vi "Tag Metadata Remove Group 01.vi"(0 "Tags Array":string[][](array[string]), 7 "Boolean Refs Array":refnum<vi>[](array[refnum]), 11 "Group Index":i32) -> (4 "Updated Tag Array":string[][](array[string]), 8 "Update Index":i32, 15 "Current Tags":string[][](array[string]))   [LabVIEW 2020]
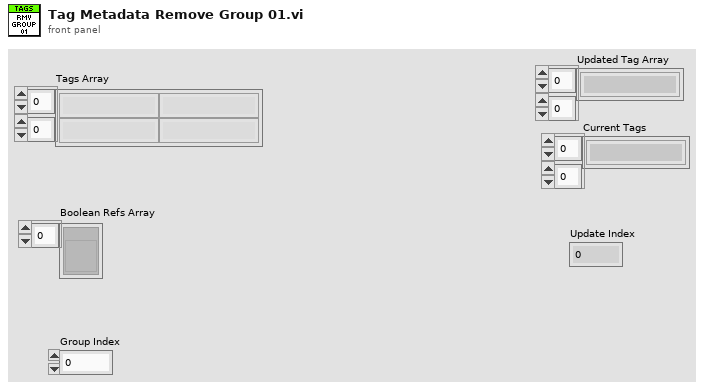
[diagram p1: front panel]
types:
  T1 = enum8{"Enabled", "Disabled", "Disabled and Grayed Out"}
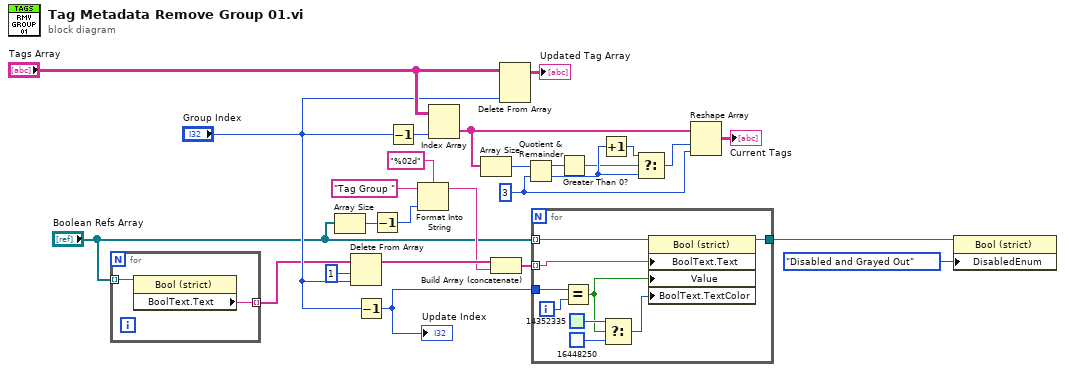
[diagram p0: block diagram]
diagram:
  w9 = 3 ("y")
  n1 = for {
    tunnel: "Boolean Refs Array" -> [w28] mode=indexing
    tunnel: [w27] -> w1 mode=indexing
    n2 = property class="Bool (strict)"(reference=w28) -> ("BoolText.Text"=w27:string)  [unwired: 1 in, 2 out]
  }
  n3 = Array Size(array="Boolean Refs Array") -> (size(s)=w22:i32)
  n4 = Delete From Array(array=w1, length=1, index="Group Index") -> (array with subset deleted=w25:string[])  [unwired: 1 out]
  n5 = Decrement(x="Group Index") -> (x-1=w7:i32)
  "Update Index" <- w7
  n6 = Decrement(x=w22) -> (x-1=w19:i32)
  n7 = Decrement(x="Group Index") -> (x-1=w8:i32)
  n8 = Format Into String(format string="%02d", initial string="Tag Group ", w19) -> (resulting string=w21:string)  [unwired: 1 in, 1 out]
  n9 = Index Array(array="Tags Array", index (col)=w8) -> (element=w10:string[])  [unwired: 1 in]
  n10 = Array Size(array=w10) -> (size(s)=w11:i32)
  n11 = Build Array (concatenate)(w25, w21) -> (w20:string[])
  n12 = Delete From Array(array="Tags Array", index (col)="Group Index") -> (array with subset deleted=→"Updated Tag Array":string[][])  [unwired: 2 in, 1 out]
  n13 = Quotient & Remainder(x=w11, y=w9) -> (x-y*floor(x/y)=w12:i32, floor(x/y)=w14:i32)
  n14 = for {
    tunnel: "Boolean Refs Array" -> [w37] mode=indexing
    tunnel: w20 -> [w34] mode=indexing
    tunnel: w7 -> [w36]
    tunnel: [w29] -> w17
    i -> [w35]
    n15 = Equal?(x=w36, y=w35) -> (x = y?=w31:bool)
    n16 = Select(t=u32 14352335 ("Color Box"), s=w31, f=u32 16448250) -> (s? t:f=w30:u32)
    n17 = property class="Bool (strict)"(reference=w37, "BoolText.Text"=w34, "Value"=w31, "BoolText.TextColor"=w30) -> (reference out=w29:refnum<vi>)  [unwired: 1 in, 1 out]
  }
  n18 = Greater Than 0?(x=w12) -> (x > 0?=w13:bool)
  n19 = Increment(x=w14) -> (x+1=w15:i32)
  n20 = Select(t=w15, s=w13, f=w14) -> (s? t:f=w16:i32)
  n21 = Reshape Array(w10, w16, w9) -> (→"Current Tags":string[][])
  n22 = property class="Bool (strict)"(reference=w17, "DisabledEnum"=T1."Disabled and Grayed Out" ("Disabled")) -> ()  [unwired: 1 in, 2 out]
